vi "Set Message Queue.vi"(8 "Error In":errorcluster, 10 "Message Queue":refnum<queue>, 11 "Process In":refnum<class "Process.lvclass">) -> (0 "Error Out":errorcluster, 3 "Process Out":refnum<class "Process.lvclass">)   [LabVIEW 2021, in "Process.lvclass"]
uses:
  Process.lvclass
  Public/Controls/Process Message.ctl
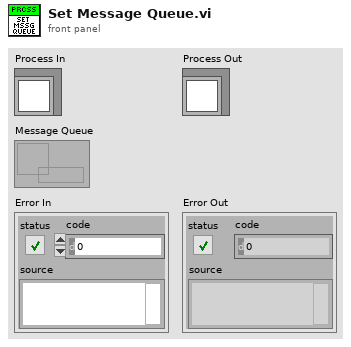
[diagram p1: front panel]
types:
  T1 = typedef "Process.lvclass/Data.ctl" = cluster{"Message Queue":refnum<queue>, "Central Message Queue":refnum<queue>}
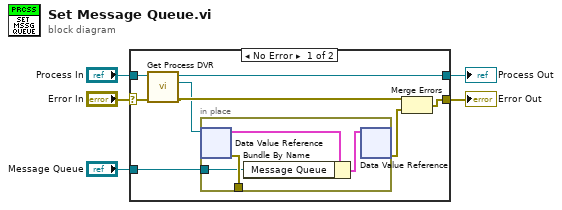
[diagram p0: block diagram]
diagram:
  n1 = case shown="No Error" "Error In" {
    selector: "Error In" -> [w9 w18]
    tunnel: [w12 w18] -> w2
    tunnel: [w8 w19] -> w5
    tunnel: "Process In" -> [w10 w19]
    tunnel: "Message Queue" -> [w11 _]
    frame No Error {
      n2 = call "Get Process DVR.vi"("Error In"=w9, "Process In"=w10) -> ("Error Out"=w7:errorcluster, "DVR"=w6:refnum<data-value>, "Process Out"=w8:refnum<class "Process.lvclass">)  [unwired: 7 in]
      n3 = in-place {
        in-place-border: [w17] -> _
        in-place-border: w11 -> [w14]
        n4 = in-place-dvr #1(w6) -> (w16:T1, w17:errorcluster)
        n5 = Bundle By Name(cluster=w16, "Message Queue"=w14) -> (w15:T1)
        n6 = in-place-dvr #1(w15) -> (w13:errorcluster)  [unwired: 1 out]
      }
      n7 = Merge Errors(w7, w13) -> (w12:errorcluster)
    }
    frame Error {
    }
  }
  "Process Out" <- w5
  "Error Out" <- w2
